vi "Periodic Tasks.vi"() -> ()   [LabVIEW 2011]
doc: "This VI runs in parallel to other tasks. It can contain as many user-defined periodic loops as you need. These can carry out PID or other sorts of timed response."
uses:
  <vilib>/Rock Robotics/SystemInterfaces/Utilities/FPGA_UtilitiesLED State.ctl
  <vilib>/Rock Robotics/SystemInterfaces/Utilities/FPGA_UtilitiesLED Source.ctl
  Robot Global Data.vi
panel:
  out "Rate":dbl
  out "Distance":dbl
  out "Angular Rate":dbl
  out "Angle":dbl
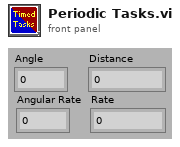
[diagram p1: front panel]
types:
  T1 = typedef "WPI_GyroDevRef.ctl" = cluster{"DevStatus":errorcluster, "Analog Module":T2, "Analog Channel":T3, "Offset":dbl, "Gain (VoltsPerDegree/Second)":dbl}
  T2 = typedef "FPGA_TypedefAnalogModule.ctl" = enum16{"Analog Module 1", "Analog Module 2"}
  T3 = typedef "FPGA_AIChannel.ctl" = enum8{"AI 1", "AI 2", "AI 3", "AI 4", "AI 5", "AI 6", "AI 7", "AI 8", "Invalid"}
  T4 = typedef "WPI_EncoderDevRef.ctl" = cluster{"DevStatus":errorcluster, "EncoderIndex":T5, "CounterIndex":T6, "DistancePerCount":dbl, "Decoding Type":T7}
  T5 = typedef "FPGA_EncoderIdx.ctl" = enum8{"Enc 0", "Enc 1", "Enc 2", "Enc 3", "Invalid"}
  T6 = typedef "FPGA_CounterCtrSystemIndex.ctl" = enum8{"Ctr 0", "Ctr 1", "Ctr 2", "Ctr 3", "Ctr 4", "Ctr 5", "Ctr 6", "Ctr 7", "Invalid"}
  T7 = typedef "WPI_EncoderType.ctl" = enum16{"1x", "2x", "4x"}
  T8 = typedef "FPGA_UtilitiesLED State.ctl" = enum16{"Off", "On", "Toggle"}
  T9 = typedef "FPGA_UtilitiesLED Source.ctl" = enum16{"User LED", "FPGA LED"}
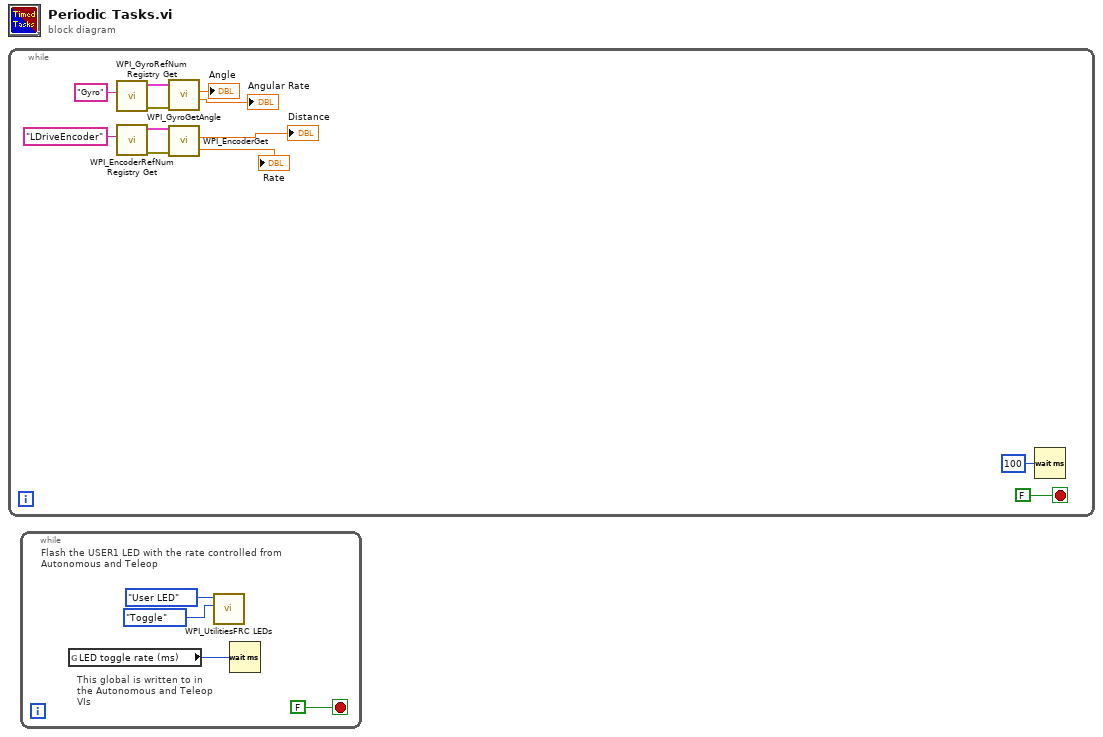
[diagram p0: block diagram]
diagram:
  n1 = while {
    stop <- FALSE stop-if-true
    n2 = call <vilib>:"WPI_GyroRefNum Registry Get.vi"("refnum name"="Gyro") -> ("error out"=w3:errorcluster, "GyroDevRef"=w4:T1)  [unwired: 9 in]
    n3 = call <vilib>:"WPI_EncoderRefNum Registry Get.vi"("refnum name"="LDriveEncoder") -> ("error out"=w1:errorcluster, "EncoderDevRef"=w2:T4)  [unwired: 9 in]
    n4 = call <vilib>:"WPI_GyroGetAngle.vi"("error in (no error)"=w3, "GyroDevRef"=w4) -> ("Angular Rate"=→"Angular Rate":dbl, "Angle"=→"Angle":dbl)  [unwired: 6 in, 2 out]
    n5 = call <vilib>:"WPI_EncoderGet.vi"("error in (no error)"=w1, "EncoderDevRef"=w2) -> ("Distance"=→"Distance":dbl, "Rate"=→"Rate":dbl)  [unwired: 4 in, 4 out]
    n6 = Wait (ms)(milliseconds to wait=u32 100) -> ()  [unwired: 1 out]
  }
  n7 = while {
    stop <- FALSE stop-if-true
    # "This global is written to in the Autonomous and Teleop VIs"
    # "Flash the USER1 LED with the rate controlled from Autonomous and Teleop"
    n8 = global read "Robot Global Data.vi" "LED toggle rate (ms)"() -> (w13:u32)
    n9 = call <vilib>:"WPI_UtilitiesFRC LEDs.vi"("State"=FPGA_UtilitiesLED_State."Toggle", "LED Type"=FPGA_UtilitiesLED_Source."User LED") -> ()  [unwired: 1 in, 9 out]
    n10 = Wait (ms)(milliseconds to wait=w13) -> ()  [unwired: 1 out]
  }
